vi "Read Self Actor Attributes.vi"(11 "Actor in":refnum<class "Actor.lvclass">) -> (2 "Self Actor Attributes":refnum<data-value>)   [LabVIEW 2020, in "jettl.lvlib" / "Actor.lvclass"]
uses:
  Actor.lvclass
  Transport/Transport.lvclass
  Actor Attributes.ctl
  jettl.lvlib
  Msg/Msg.lvclass
  Msgs.ctl
  Unified Layer.ctl
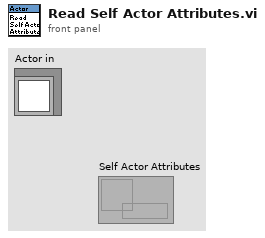
[diagram p1: front panel]
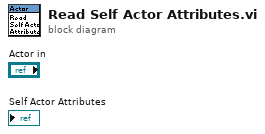
[diagram p0: block diagram]
diagram:
